vi "SetSDAT.vi"(8 "error in (no error)":errorcluster) -> (0 "error out":errorcluster)   [LabVIEW 2015, in "ESLSCDLL.lvlib"]
uses:
  ESLSCDLL.lvlib
  Globals.vi
  ESLSCDLL.dll
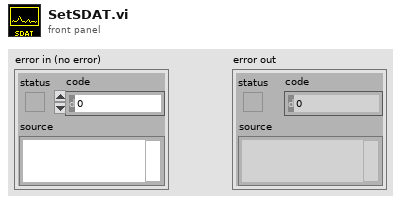
[diagram p1: front panel]
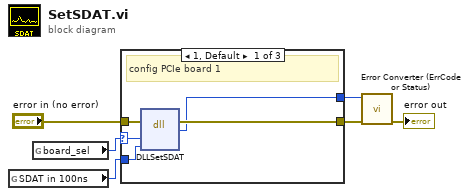
[diagram p0: block diagram]
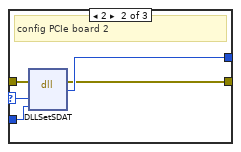
[diagram p2: hidden frame]
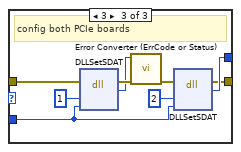
[diagram p3: hidden frame]
diagram:
  n1 = global read "Globals.vi" "SDAT in 100ns"() -> (w1:u32)
  n2 = global read "Globals.vi" "board_sel"() -> (w2:u32)
  n3 = case shown="1, Default" w2 {
    selector: w2 -> [w11 w15 _]
    tunnel: "error in (no error)" -> [w10 w16 w25]
    tunnel: [w9 w12 w19] -> w5
    tunnel: [w8 w13 w20] -> w3
    tunnel: w1 -> [w7 w14 w21]
    frame 1, Default {
      # "config PCIe board 1"
      n4 = dll-call lib="C:/ENTW/PCIE/LV64/board.vis/ESLSCDLL.dll" fn="DLLSetSDAT" ("lwlscdll.dll:DLLSetTemp")(error in=w10, "drv"=w11, "sdat_in_100ns"=w7) -> (error out=w9:errorcluster, "es_status_codes"=w8:i32)  [unwired: 4 in, 1 out]
    }
    frame 2 {
      # "config PCIe board 2"
      n5 = dll-call lib="C:/ENTW/PCIE/LV64/board.vis/ESLSCDLL.dll" fn="DLLSetSDAT" ("lwlscdll.dll:DLLSetTemp")(error in=w16, "drv"=w15, "sdat_in_100ns"=w14) -> (error out=w12:errorcluster, "es_status_codes"=w13:i32)  [unwired: 4 in, 1 out]
    }
    frame 3 {
      # "config both PCIe boards"
      n6 = dll-call lib="C:/ENTW/PCIE/LV64/board.vis/ESLSCDLL.dll" fn="DLLSetSDAT" ("lwlscdll.dll:DLLSetTemp")(error in=w25, "drv"=u32 1, "sdat_in_100ns"=w21) -> (error out=w18:errorcluster, "es_status_codes"=w17:i32)  [unwired: 4 in, 1 out]
      n7 = call "Error Converter (ErrCode or Status).vi"("error in (no error)"=w18, "error code"=w17) -> ("error out"=w23:errorcluster)  [unwired: 9 in]
      n8 = dll-call lib="C:/ENTW/PCIE/LV64/board.vis/ESLSCDLL.dll" fn="DLLSetSDAT" ("lwlscdll.dll:DLLSetTemp")(error in=w23, "drv"=u32 2, "sdat_in_100ns"=w21) -> (error out=w19:errorcluster, "es_status_codes"=w20:i32)  [unwired: 4 in, 1 out]
    }
  }
  n9 = call "Error Converter (ErrCode or Status).vi"("error in (no error)"=w5, "error code"=w3) -> ("error out"=→"error out":errorcluster)  [unwired: 9 in]
